vi "Assert Message.vi"(8 "error in (no error)":errorcluster, 9 "Mock":refnum<class "LMock Mock.lvclass">, 10 "Message":string, 11 "LUnit Test Case In":refnum<class "Test Case.lvclass">) -> (0 "error out":errorcluster, 3 "LUnit Test Case Out":refnum<class "Test Case.lvclass">)   [LabVIEW 2020, in "Expectation Test.lvclass"]
uses:
  Expectation Test.lvclass
  source/Framework/Mock/LMock Mock.lvclass
  <vilib>/Astemes/LUnit/Test Case.lvclass
  <vilib>/Astemes/LUnit/Test Case.lvclass/Test Case.ctl
  <vilib>/Astemes/LUnit/Append Pass Result.vi
  <vilib>/Astemes/LUnit/Append Fail Result.vi
  <vilib>/Astemes/LUnit/Describe Comparison.vi
  <vilib>/Astemes/LUnit/Compare Variants.vi
  <vilib>/Astemes/LUnit/Variant to string.vi
  <vilib>/Utility/Data Type/Get Type Information.vi
  <vilib>/Utility/LVClass/Get LV Class Name.vi
  Expectation Test.lvclass/Expectation Test.ctl
  c92b63b2-ed3c-4a03-a3e4-e829322695b9.vi
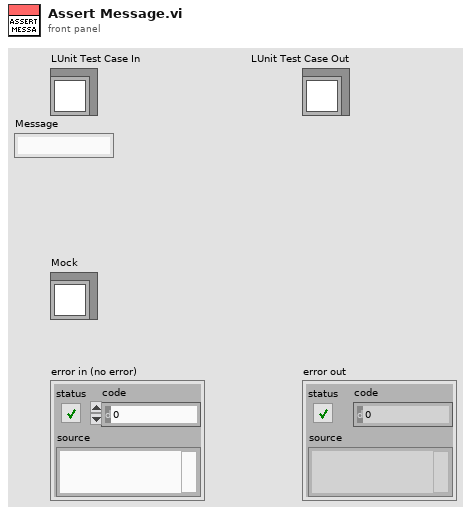
[diagram p1: front panel]
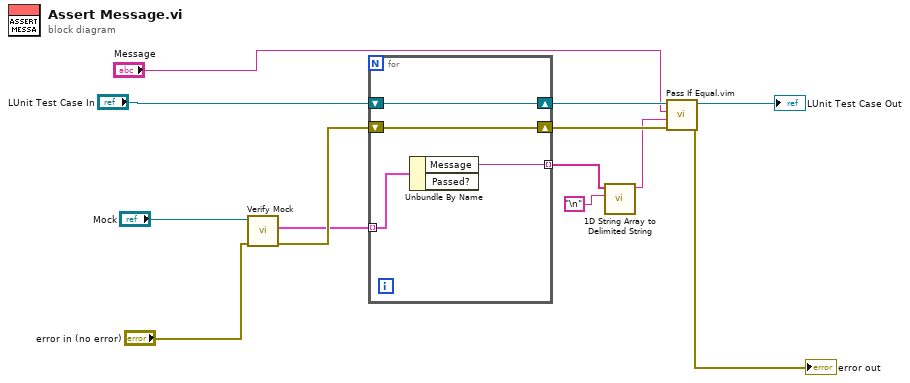
[diagram p0: block diagram]
diagram:
  n1 = call-dynamic "Verify Mock.vi"("error in (no error)"="error in (no error)", "Mock In"="Mock") -> ("error out"=w10:errorcluster, "Results"=w8:cluster{"Passed?":bool, "Message":string}[])  [unwired: 7 in, 1 out]
  n2 = for {
    shift-right: [w17] -> w13
    shift-left: w10 -> [w17]
    shift-right: [w16] -> w6
    shift-left: "LUnit Test Case In" -> [w16]
    tunnel: w8 -> [w15] mode=indexing
    tunnel: [w14] -> w4 mode=indexing
    n3 = Unbundle By Name(w15) -> ("Message"=w14:string)  [unwired: 1 out]
  }
  n4 = call <vilib>:"1D String Array to Delimited String.vi"("delimiter"="\n", "string array"=w4) -> ("delimited string"=w2:string)  [unwired: 9 in]
  n5 = call "Pass If Equal.vim"("error in (no error)"=w13, "Actual"=w2, "Expected"="Message", "LUnit Test Case In"=w6) -> ("error out"=→"error out":errorcluster, "LUnit Test Case Out"=→"LUnit Test Case Out":refnum<class "Test Case.lvclass">)  [unwired: 6 in]
